vi "Calculate V2C.vi"(9 "Tcal_Chamber":dbl, 10 "Voltage In":dbl format="%_6g", 11 "Calibration Coefficients":T1={"CalFile Used"=path "", "TYPE"="", "DATE"="", "Humidity"=0.0, "Chamber Temp"=0.0, "CO2_calgas"=nan, "V_(RA,5mA)"=nan, "V_(RA,15mA)"=nan, "mI"=nan, "V_0d_ImA (actual)"=nan, "V_6d_ImA (actual)"=nan, "I_span"=nan, "DAC"=0, "A"=nan, "B"=nan, "C"=nan, "D"=nan, "V6d"=nan, "A'"=0.0, "B'"=0.0, "C'"=0.0, "D'"=0.0, "V0d"=0.0, "CalDate"="", "CalTime"="", "duration"=0.0, "Detector Channel"="", "a2"=nan, "a3"=nan, "a4"=nan, "a5"=nan, "b2"=nan, "c2"=nan, "b3"=nan, "c3"=nan, "b4"=nan, "c4"=nan, "b5"=nan, "c5"=nan, "a7"=nan, "a8"=nan, "a9"=nan, "a10"=nan, "b7"=nan, "b8"=nan, "b9"=nan, "b10"=nan, "c7"=nan, "c8"=nan, "c9"=nan, "c10"=nan, "cal_offs_adj"=0.0, "cal_gain_adj"=1.0, "C6d"=nan, "C0d"=0.0, "Cal_currernt"=nan, "C2V"=0, "V2C"=0, "Zero Date"="", "Zero Time"="", "Number of Zeroes"=0, "V_(()d, average)"=nan, "V_offs "=0.0, "G_adj"=1.0, "Pump Flow Rate"=0, "Zero Required? "=FALSE, "Calibrate Required?"=FALSE, "cal_utc"=0.0, "zero_utc"=0.0, "Elapsed Time"=0.0, "PCB"="", "m0"=0.0, "b0"=0.0} {"Elapsed Time" format="%<%H:%M:%S>t"; "Pump Flow Rate" format="%0d"; "Number of Zeroes" format="%0d"; "V2C" format="%0d"; "C2V" format="%0d"; "duration" format="%<%H:%M:%S>t"; "DAC" format="%03x"; "mI" format="%.3g"; "V_(RA,15mA)" format="%0.4f"; "V_(RA,5mA)" format="%0.4f"; "Chamber Temp" format="%.1f"; "Humidity" format="%.1f"}) -> (0 "C'":dbl format="%_6g", 1 "B'":dbl format="%_6g", 2 "A'":dbl format="%_6g", 3 "CO2 Out":dbl format="%_6g", 4 "D'":dbl format="%_6g")   [LabVIEW 2016]
uses:
  Controls/Calibration Coefficients.ctl
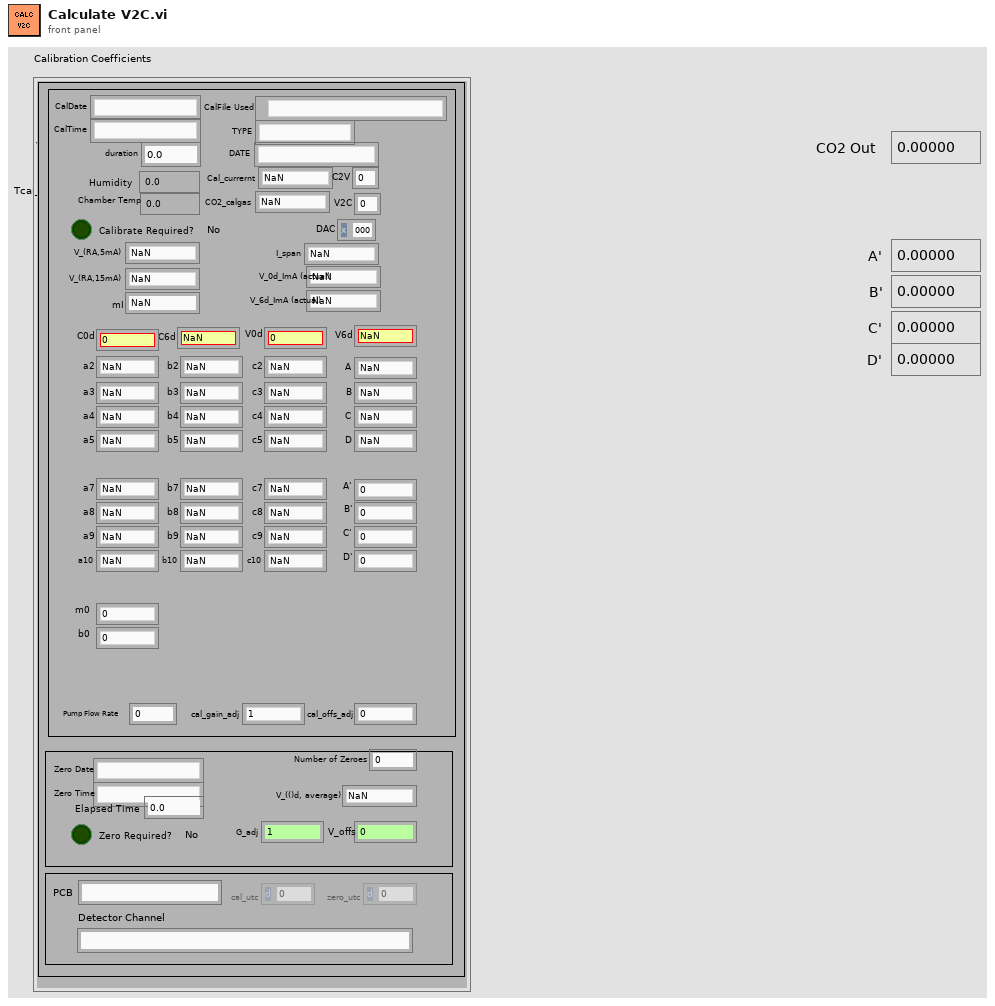
[diagram p1: front panel]
types:
  T1 = typedef "Calibration Coefficients.ctl" = cluster{"CalFile Used":path, "TYPE":string, "DATE":string, "Humidity":sgl, "Chamber Temp":dbl, "CO2_calgas":dbl, "V_(RA,5mA)":dbl, "V_(RA,15mA)":dbl, "mI":dbl, "V_0d_ImA (actual)":dbl, "V_6d_ImA (actual)":dbl, "I_span":dbl, "DAC":u16, "A":dbl, "B":dbl, "C":dbl, "D":dbl, "V6d":dbl, "A'":dbl, "B'":dbl, "C'":dbl, "D'":dbl, "V0d":dbl, "CalDate":string, "CalTime":string, "duration":dbl, "Detector Channel":string, "a2":dbl, "a3":dbl, "a4":dbl, "a5":dbl, "b2":dbl, "c2":dbl, "b3":dbl, "c3":dbl, "b4":dbl, "c4":dbl, "b5":dbl, "c5":dbl, "a7":dbl, "a8":dbl, "a9":dbl, "a10":dbl, "b7":dbl, "b8":dbl, "b9":dbl, "b10":dbl, "c7":dbl, "c8":dbl, "c9":dbl, "c10":dbl, "cal_offs_adj":dbl, "cal_gain_adj":dbl, "C6d":dbl, "C0d":dbl, "Cal_currernt":dbl, "C2V":u16, "V2C":u16, "Zero Date":string, "Zero Time":string, "Number of Zeroes":u16, "V_(()d, average)":dbl, "V_offs ":dbl, "G_adj":dbl, "Pump Flow Rate":u16, "Zero Required? ":bool, "Calibrate Required?":bool, "cal_utc":dbl, "zero_utc":dbl, "Elapsed Time":dbl, "PCB":string, "m0":dbl, "b0":dbl}
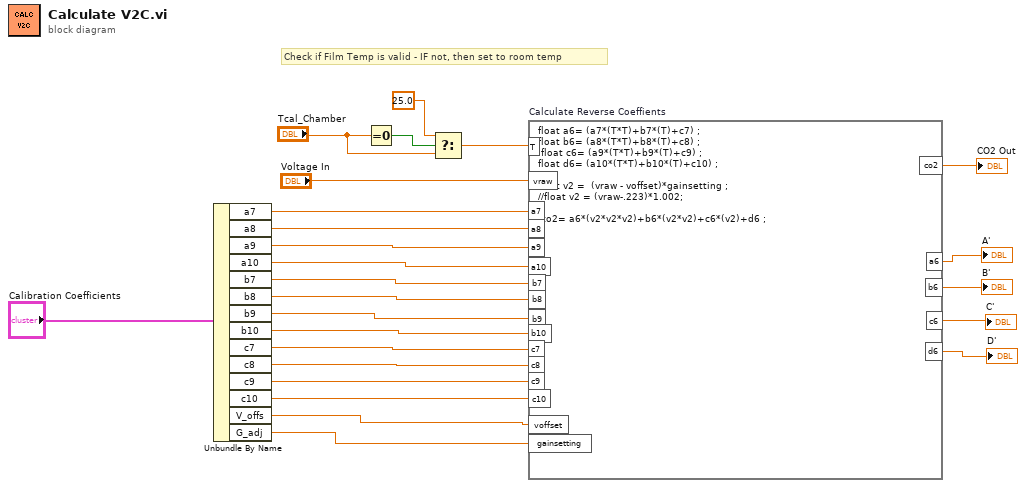
[diagram p0: block diagram]
diagram:
  # "Check if Film Temp is valid - IF not, then set to room temp"
  n1 = Unbundle By Name("Calibration Coefficients") -> ("a7"=w14:dbl, "a8"=w15:dbl, "a9"=w16:dbl, "a10"=w17:dbl, "b7"=w18:dbl, "b8"=w19:dbl, "b9"=w20:dbl, "b10"=w21:dbl, "c7"=w22:dbl, "c8"=w23:dbl, "c9"=w24:dbl, "c10"=w25:dbl, "V_offs"=w7:dbl, "G_adj"=w6:dbl)
  n2 = Equal To 0?(x="Tcal_Chamber") -> (x = 0?=w4:bool)
  n3 = Select(t=25.0, s=w4, f="Tcal_Chamber") -> (s? t:f=w2:dbl)
  n4 = formula code="float\ta6=\t(a7*(T*T)+b7*(T)+c7)\t;\nfloat\tb6=\t(a8*(T*T)+b8*(T)+c8)\t;\n\tfloat c6=\t(a9*(T*T)+b9*(T)+c9)\t;\nfloat\td6=\t(a10*(T*T)+b10*(T)+c10)\t;\n\t\t\t\nfloat\tv2 = \t(vraw - voffset)*gainsetting\t;\n//float v2 = (vraw-.223)*1.002;\n\t\t\n\tco2=\ta6*(v2*v2*v2)+b6*(v2*v2)+c6*(v2)+d6\t;" "Calculate Reverse Coeffients"("vraw"="Voltage In", "T"=w2, "a7"=w14, "a8"=w15, "a9"=w16, "a10"=w17, "b7"=w18, "b8"=w19, "b9"=w20, "b10"=w21, "c7"=w22, "c8"=w23, "c9"=w24, "c10"=w25, "voffset"=w7, "gainsetting"=w6) -> ("co2"=→"CO2 Out":dbl, "a6"=→"A'":dbl, "b6"=→"B'":dbl, "c6"=→"C'":dbl, "d6"=→"D'":dbl)
